vi "SingleWellUpdater.vi"(9 "Temps":dbl[][](graph)=array384x528[202752 elements], 10 "Well Coordinates":T2[](array[typedef]) {"Y" format="%.2f"; "X" format="%.2f"}, 11 "Last Mouse Position":cluster{"X":i32, "Y":i32}) -> (1 "Well idx":i32, 2 "ROI Descriptor":T1 {"Contours"."Type" items=["No Selection", "Point", "Line", "Rectangle", "Oval", "Polygon", "Freehand Region", "Annulus", "Unused2", "Unused3", "Broken Line", "Freehand Line", "Rotated Rectangle"]}, 3 "State out":string)   [LabVIEW 2022 SP3]
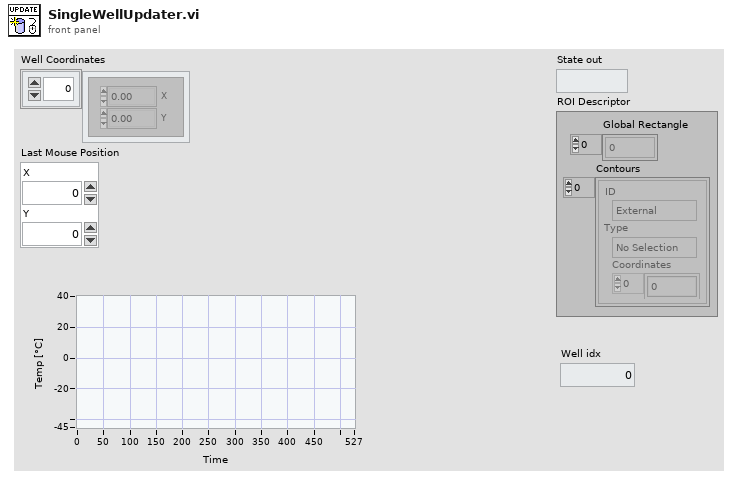
[diagram p1: front panel]
types:
  T1 = typedef "ROI Descriptor" = cluster{"Global Rectangle":i32[], "Contours":cluster{"ID":enum32{"External", "Internal"}, "Type":u32, "Coordinates":i32[]}[]}
  T2 = typedef "IMAQ Point" = cluster{"X":sgl, "Y":sgl}
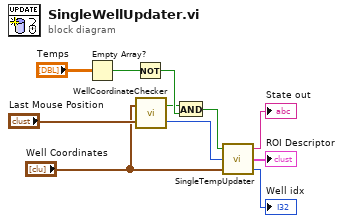
[diagram p0: block diagram]
diagram:
  n1 = Empty Array?(array="Temps") -> (empty?=w5:bool)
  n2 = Not(x=w5) -> (.not. x?=w4:bool)
  n3 = call "WellCoordinateChecker.vi"("Last Mouse Position"="Last Mouse Position", "Well Coordinates"="Well Coordinates") -> ("Well Idx"=w9:i32, "Valid Point?"=w3:bool)
  n4 = And(x=w3, y=w4) -> (x .and. y?=w2:bool)
  n5 = call "SingleTempUpdater.vi"("Well Coordinates"="Well Coordinates", "Well idx"=w9, "Valid Point?"=w2) -> ("Well idx"=→"Well idx":i32, "ROI Descriptor"=→"ROI Descriptor":T1, "State out"=→"State out":string)
